vi "生产者消费者架构的串口高速数据采集.vi"() -> ()   [LabVIEW 2013]
uses:
  <vilib>/Instr/_visa.llb/VISA Configure Serial Port (Instr).vi
panel:
  out "运行时间":string caption="开始时间："
  out "开始时间":string caption="开始时间："
  in  "采样周期（ms）":u32=10
  out "温度曲线":dbl(graph)
  out "温度值":dbl format="%.2g"
  in  "端口":refnum<visa-resource-name> caption="串口号"
  in  "停止按钮":bool
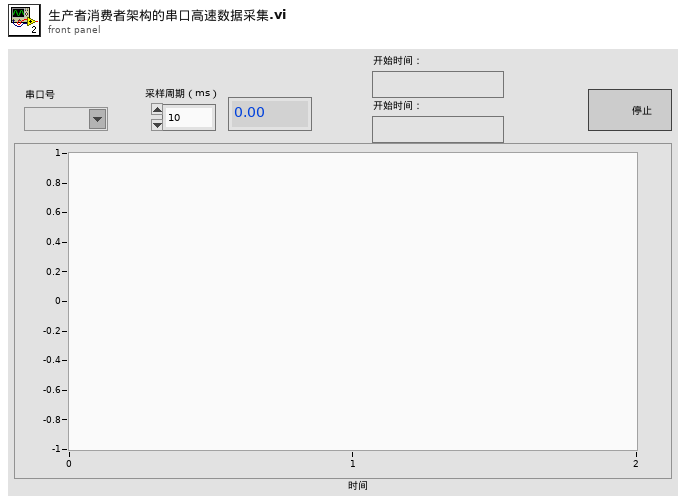
[diagram p1: front panel]
types:
  T1 = enum16{"open", "replace", "create", "open or create", "replace or create", "replace or create with confirmation"}
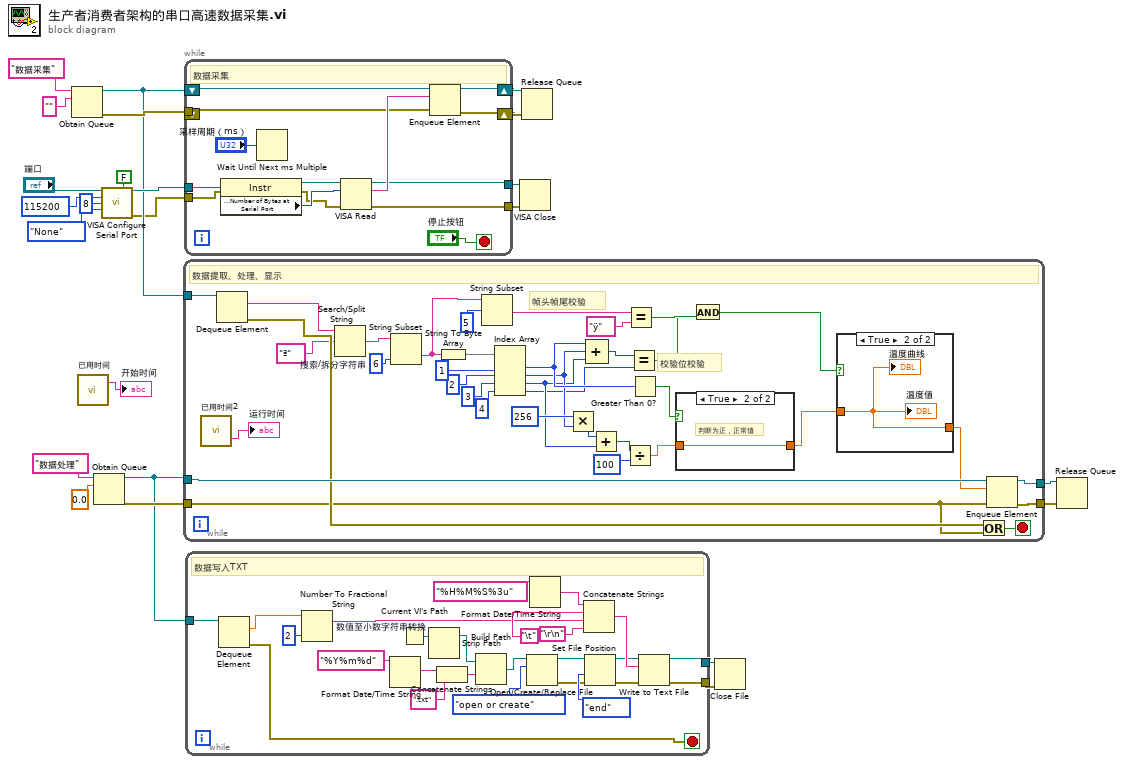
[diagram p0: block diagram]
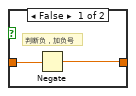
[diagram p3: hidden frame]
diagram:
  n1 = Obtain Queue(name (unnamed)="数据采集" ("名称（未命名）"), element data type="") -> (queue out=w6:refnum<queue>, error out=w8:errorcluster)  [unwired: 3 in, 1 out]
  n2 = call "已用时间"() -> ("Present Text"=→"开始时间":string)  [unwired: 12 in, 7 out]
  n3 = Obtain Queue(name (unnamed)="数据处理" ("名称（未命名）"), element data type=0.0) -> (queue out=w13:refnum<queue>, error out=w16:errorcluster)  [unwired: 3 in, 1 out]
  n4 = call-poly "VISA Configure Serial Port"("VISA resource name"="端口", "Enable Termination\nChar (T)"=FALSE ("Enable Termination\nChar (T)"), "baud rate (9600)"=u32 115200, "data bits (8)"=u16 8, "parity (0:none)"=enum16{"None", "Odd", "Even", "Mark", "Space"}."None") -> ("VISA resource name out"=w18:refnum<visa-resource-name>, "error out"=w3:errorcluster)  [unwired: 9 in]
  n5 = while {
    tunnel: w6 -> [w61]
    tunnel: w13 -> [w35]
    tunnel: w16 -> [w31]
    tunnel: [w34] -> w15
    tunnel: [w33] -> w14
    stop <- w30 stop-if-true
    # "帧头帧尾校验"
    # "校验位校验"
    # "数据提取、处理、显示"
    n6 = call "已用时间2"() -> ("Elapsed Time Text"=→"运行时间":string)  [unwired: 12 in, 7 out]
    n7 = Dequeue Element(queue=w61) -> (element=w36:string, error out=w32:errorcluster)  [unwired: 2 in, 2 out]
    n8 = Search/Split String "搜索/拆分字符串"(string=w36, search string/char (-)="ª" ("y")) -> (match + rest of string=w38:string)  [unwired: 1 in, 2 out]
    n9 = String Subset(string=w38, length (rest)=6 ("长度（剩余）")) -> (substring=w37:string)  [unwired: 1 in]
    n10 = String To Byte Array ("字符串至字节数组转换")(string=w37) -> (unsigned byte array=w56:u8[])
    n11 = String Subset(string=w37, offset (0)=5 ("长度（剩余）")) -> (substring=w43:string)  [unwired: 1 in]
    n12 = Index Array(array=w56, index #1=1 ("索引"), index #2=2 ("索引 2"), index #3=3 ("索引 3"), index #4=4 ("索引")) -> (element #1=w49:u8, element #2=w48:u8, element #3=w47:u8, element #4=w45:u8)
    n13 = Multiply(x=u32 256, y=w48) -> (x*y=w59:u32)
    n14 = Compound Arithmetic op=ADD(w49, w48, w47) -> (w46:u8)
    n15 = Add(x=w59, y=w47) -> (x+y=w58:u32)
    n16 = Divide(x=w58, y=u32 100) -> (x/y=w51:dbl)
    n17 = Equal?(x=w43, y="ÿ") -> (x = y?=w41:bool)
    n18 = Equal?(x=w46, y=w45) -> (x = y?=w40:bool)
    n19 = Greater Than 0?(x=w49) -> (x > 0?=w52:bool)
    n20 = case shown="True" w52 {
      tunnel: w51 -> [w64 w65]
      tunnel: [w63 w65] -> w27
      frame False {
        # "判断负，加负号"
        n21 = Negate(x=w64) -> (-x=w63:dbl)
      }
      frame True {
        # "判断为正，正常值"
      }
    }
    n22 = And(x=w41, y=w40) -> (x .and. y?=w28:bool)
    n23 = case shown="True" w28 {
      tunnel: w27 -> [_ w62]
      tunnel: [_ w62] -> w26
      frame False {
      }
      frame True {
        "温度值" <- w62
        "温度曲线" <- w62
      }
    }
    n24 = Or(x=w32, y=w31) -> (x .or. y?=w30:bool)
    n25 = Enqueue Element(queue=w35, element=w26, error in (no error)=w31) -> (queue out=w34:refnum<queue>, error out=w33:errorcluster)  [unwired: 1 in, 1 out]
  }
  n26 = while {
    tunnel: w18 -> [w77]
    tunnel: [w74] -> w9
    tunnel: w8 -> [w73]
    shift-right: [w72] -> w7
    shift-left: _ -> [_]
    shift-right: [w70] -> w5
    shift-left: w6 -> [w71]
    tunnel: w3 -> [w68]
    tunnel: [w66] -> w2
    stop <- "停止按钮" stop-if-true
    # "数据采集"
    n27 = property class="Instr"(reference=w77, error in=w68) -> (reference out=w76:refnum<visa-resource-name>, error out=w67:errorcluster, "Serial Settings:Number of Bytes at Serial Port"=w75:u32)
    n28 = Wait Until Next ms Multiple(millisecond multiple="采样周期（ms）") -> ()  [unwired: 1 out]
    n29 = VISA Read(VISA resource name=w76, byte count=w75, error in (no error)=w67) -> (VISA resource name out=w74:refnum<visa-resource-name>, read buffer=w78:string, error out=w66:errorcluster)  [unwired: 1 out]
    n30 = Enqueue Element(queue=w71, element=w78, error in (no error)=w73) -> (queue out=w70:refnum<queue>, error out=w72:errorcluster)  [unwired: 1 in, 1 out]
  }
  n31 = while {
    tunnel: w13 -> [w104]
    tunnel: [w81] -> w12
    tunnel: [w80] -> w1
    stop <- w103 stop-if-true
    # "数据写入TXT"
    n32 = Dequeue Element(queue=w104) -> (element=w82:dbl, error out=w103:errorcluster)  [unwired: 2 in, 2 out]
    n33 = Number To Fractional String "数值至小数字符串转换"(number=w82, precision (6)=i16 2 ("精度(6)")) -> (F-format string=w83:string)  [unwired: 2 in]
    n34 = Format Date/Time String(time format string (%c)="%Y%m%d" ("时间格式字符串(%c)")) -> (date/time string=w85:string)  [unwired: 2 in]
    n35 = Current VI's Path() -> (path=w92:path)
    n36 = Strip Path(path=w92) -> (stripped path=w91:path)  [unwired: 1 out]
    n37 = Concatenate Strings(w85, ".txt" ("名称或相对路径")) -> (w101:string)
    n38 = Build Path(base path=w91, name or relative path=w101) -> (appended path=w96:path)
    n39 = Open/Create/Replace File(file path (use dialog)=w96, operation (0:open)=T1."open or create" ("操作(0:open)")) -> (refnum out=w97:refnum<file>, error out=w98:errorcluster)  [unwired: 4 in, 1 out]
    n40 = Format Date/Time String(time format string (%c)="%H%M%S%3u" ("时间格式字符串(%c)")) -> (date/time string=w87:string)  [unwired: 2 in]
    n41 = Concatenate Strings(w87, "\t", w83, "\r\n") -> (w94:string)
    n42 = Set File Position(refnum=w97, from (0:start)=enum16{"start", "end", "current"}."end" ("自（0:起始）"), error in=w98) -> (refnum out=w90:refnum<file>, error out=w89:errorcluster)  [unwired: 1 in]
    n43 = Write to Text File(file (use dialog)=w90, text=w94, error in=w89) -> (refnum out=w81:refnum<file>, error out=w80:errorcluster)  [unwired: 1 in, 1 out]
  }
  n44 = VISA Close(VISA resource name=w9, error in (no error)=w2) -> ()  [unwired: 1 out]
  n45 = Release Queue(queue=w5, error in (no error)=w7) -> ()  [unwired: 1 in, 3 out]
  n46 = Close File(refnum=w12, error in=w1) -> ()  [unwired: 2 out]
  n47 = Release Queue(queue=w15, error in (no error)=w14) -> ()  [unwired: 1 in, 3 out]
